vi "Balance_Sweep_Sever.vi"(6 "Mode":bool, 7 "Filename":string, 8 "error in":errorcluster, 9 "Sample Freq (Hz)":dbl=20000.0, 10 "Stop Angle (deg)":dbl=-2.0, 11 "Measurement Time (ms)":u32) -> (0 "error out":errorcluster)   [LabVIEW 2011]
uses:
  Gen Trav/Trav_mode.ctl
  Globals/Trav_pos_global.vi
  Globals/Meas_global.vi
  Controls/Post_Process.ctl
  <userlib>/LV-Link3/PolySubVIs/DtCreateAinChan.vi
  <userlib>/LV-Link3/PolySubVIs/DtOLReadMultiple2D.vi
  <userlib>/LV-Link3/PolySubVIs/DtOLTimingSetInput.vi
  Controls/Live Balance Data.ctl
panel:
  out "status":bool=TRUE
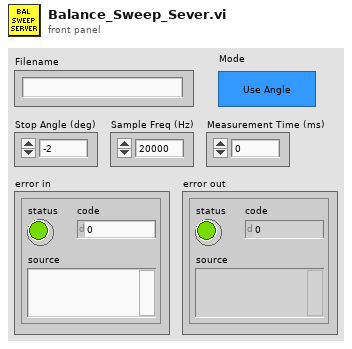
[diagram p1: front panel]
types:
  T1 = typedef "Post_Process.ctl" = enum16{"Take New Data", "Post Process Raw Data File"}
  T2 = typedef "Trav_mode.ctl" = enum16{"Move traverse", "Read traverse position", "Teach Position"}
  T3 = typedef "Live Balance Data.ctl" = cluster{"AS Freq (Hz)":dbl, "Time (s)":dbl[], "Pressure 2 (V)":dbl[], "Pressure 3 (V)":dbl[], "Wind Speed (m/s)":dbl[], "Balance AS Freq (Hz)":dbl[], "Live Angle (deg)":dbl[], "Live Angle An(deg)":dbl[], "Balance Loads":cluster{"Lift (%)":dbl[], "Lift (N)":dbl[], "Pitch (%)":dbl[], "Pitch (Nm)":dbl[], "Drag (%)":dbl[], "Drag (N)":dbl[], "Side (%)":dbl[], "Side (N)":dbl[], "Yaw (%)":dbl[], "Yaw (Nm)":dbl[], "Roll (%)":dbl[], "Roll (Nm)":dbl[]}, "Pressure 1 (V)":dbl[], "Pressure SJ (V)":dbl[]}
  T4 = enum16{"big-endian, network order", "native, host order", "little-endian"}
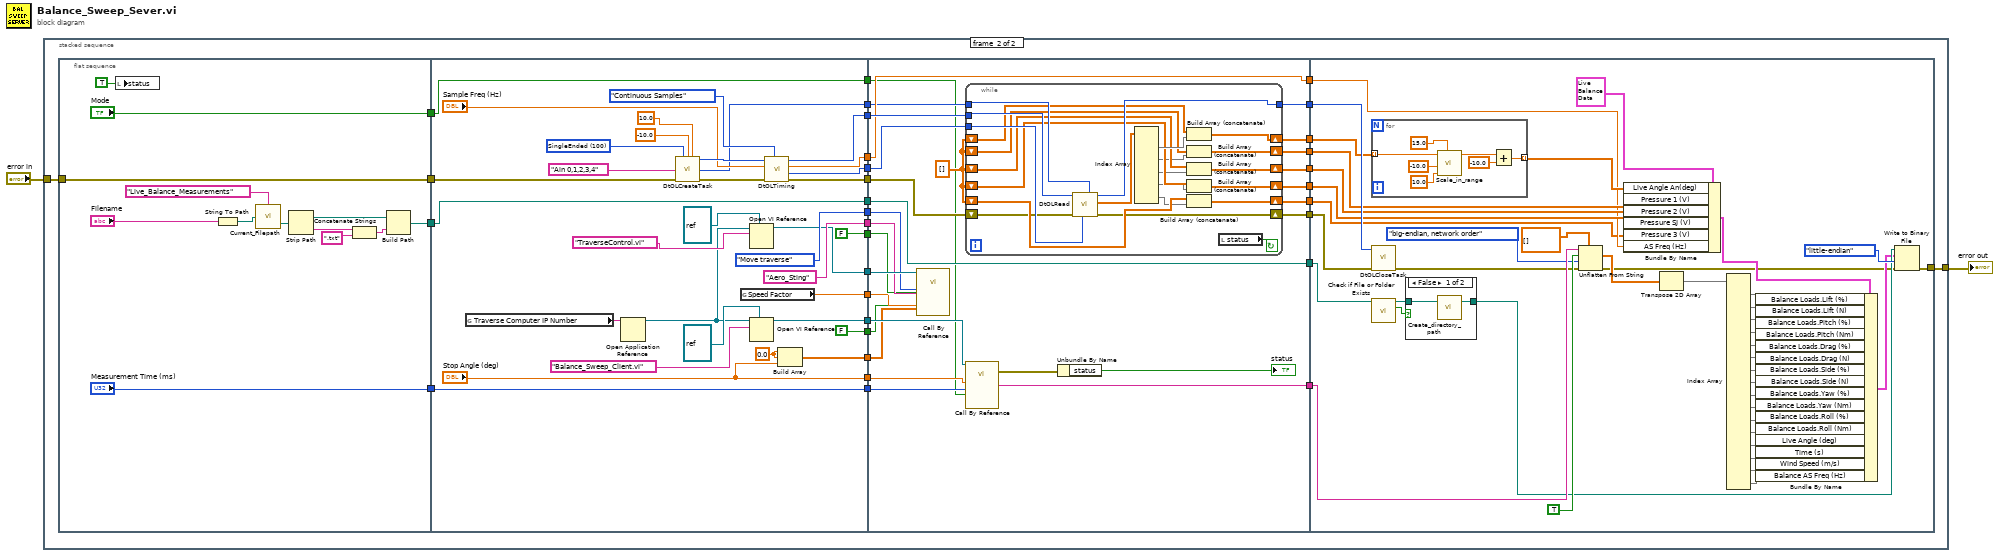
[diagram p0: block diagram]
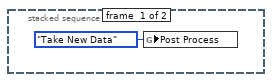
[diagram p2: hidden frame]
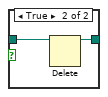
[diagram p3: hidden frame]
diagram:
  n1 = stacked-sequence {
    tunnel: [_ w12] -> w2
    tunnel: "error in" -> [_ w8]
    frame #0 {
      n2 = global write "Meas_global.vi" "Post Process"(Post_Process."Take New Data" ("Post Process")) -> ()
    }
    frame #1 {
      n3 = flat-sequence {
        tunnel: [w45] -> w36
        tunnel: [w39] -> w11
        tunnel: w8 -> [w39]
        tunnel: ["Measurement Time (ms)"] -> w7
        tunnel: ["Mode"] -> w4
        tunnel: [FALSE ("Route Checking?")] -> w35
        tunnel: [Trav_mode."Move traverse" ("Mode")] -> w34
        tunnel: ["Aero_Sting" ("Traverse name")] -> w33
        tunnel: [w78] -> w32
        tunnel: [w76] -> w31
        tunnel: ["Stop Angle (deg)"] -> w30
        tunnel: [w73] -> w29
        tunnel: [w68] -> w28
        tunnel: w36 -> [w73]
        tunnel: [w67] -> w25
        tunnel: [FALSE ("Backlash Compensation?")] -> w24
        tunnel: [w58] -> w23
        tunnel: [w57] -> w22
        tunnel: [w56] -> w20
        tunnel: [w55] -> w19
        tunnel: w11 -> [w54]
        tunnel: [w52] -> w10
        tunnel: w7 -> [w51]
        tunnel: [w51] -> w6
        tunnel: [w50] -> w5
        tunnel: w4 -> [w50]
        tunnel: w35 -> [w102]
        tunnel: w34 -> [w103]
        tunnel: w33 -> [w105]
        tunnel: w32 -> [w104]
        tunnel: w31 -> [w110]
        tunnel: [w109] -> w27
        tunnel: w30 -> [w108]
        tunnel: [w107] -> w26
        tunnel: w29 -> [w107]
        tunnel: w28 -> [w106]
        tunnel: w25 -> [w101]
        tunnel: w24 -> [w100]
        tunnel: w23 -> [w99]
        tunnel: w22 -> [w98]
        tunnel: [w97] -> w21
        tunnel: w20 -> [w97]
        tunnel: w19 -> [w96]
        tunnel: [w95] -> w18
        tunnel: [w93] -> w17
        tunnel: [w92] -> w16
        tunnel: [w91] -> w15
        tunnel: [w90] -> w14
        tunnel: [w88] -> w13
        tunnel: w10 -> [w86]
        tunnel: [w85] -> w9
        tunnel: w6 -> [w84]
        tunnel: w5 -> [w83]
        tunnel: w27 -> [w170]
        tunnel: w26 -> [w175]
        tunnel: w21 -> [w139]
        tunnel: w18 -> [w166]
        tunnel: w17 -> [w141]
        tunnel: w16 -> [w144]
        tunnel: w15 -> [w143]
        tunnel: w14 -> [w142]
        tunnel: w13 -> [w138]
        tunnel: [w137] -> w12
        tunnel: w9 -> [w136]
        frame #0 {
          n4 = local write "status"(TRUE ("status")) -> ()
          n5 = String To Path(string="Filename") -> (path=w47:path)
          n6 = call "Current_Filepath.vi"("Filename in"=w47, "Data Type"="Live_Balance_Measurements") -> ("Filename Out"=w48:path)  [unwired: 1 out]
          n7 = Strip Path(path=w48) -> (stripped path=w41:path, name=w44:string)
          n8 = Concatenate Strings(w44, ".txt" ("string")) -> (w42:string)
          n9 = Build Path(base path=w41, name or relative path=w42) -> (appended path=w45:path)
        }
        frame #1 {
          w62 = 100 items=["SingleEnded"=100, "Differential"=101] ("Channel Type")
          w82 = 0.0
          n10 = global read "Trav_pos_global.vi" "Traverse Computer IP Number"() -> (w72:string)
          n11 = Open Application Reference(11:w72) -> (3:w69:refnum<vi>)  [unwired: 3 in, 1 out]
          n12 = call-poly <userlib>:"DtOLCreateTask.vi"("Channel Type"=w62, "Range Min"=-10.0, "Range Max"=10.0, "Channel"="Ain 0,1,2,3,4", "error in (no error)"=w54) -> ("Task out"=w61:i32, "Actual Number of Channels"=w55:u32, "error out"=w53:errorcluster)  [unwired: 8 in]
          n13 = global read "Trav_pos_global.vi" "Speed Factor"() -> (w67:dbl)
          n14 = Open VI Reference(type specifier VI Refnum (for type only)=refnum<vi> refnum, application reference (local)=w69, vi path="TraverseControl.vi" ("Traverse name")) -> (vi reference=w68:refnum<vi>)  [unwired: 3 in, 1 out]
          n15 = Open VI Reference(type specifier VI Refnum (for type only)=refnum<vi> refnum, application reference (local)=w69, vi path="Balance_Sweep_Client.vi" ("Traverse name")) -> (vi reference=w76:refnum<vi>)  [unwired: 3 in, 1 out]
          n16 = call-poly <userlib>:"DtOLTiming.vi"("Sample Mode"=enum16{"Finite Samples", "Continuous Samples"}."Continuous Samples", "error in (no error)"=w53, "Sample Freq (Hz)"="Sample Freq (Hz)", "Task in"=w61) -> ("error out"=w52:errorcluster, "Buffer Size"=w58:u32, "Actual Sample Freq"=w56:dbl, "Task out"=w57:i32)  [unwired: 4 in]
          n17 = Build Array(w82, w82, "Stop Angle (deg)") -> (w78:dbl[])
        }
        frame #2 {
          w89 = dbl[] []
          n18 = call-by-ref "?"(reference=w106, "Mode"=w103, "Route Checking?"=w102, "Traverse Name"=w105, "Position input XYZ"=w104, "Speed Factor"=w101, "Backlash Compensation?"=w100) -> ()  [unwired: 9 in, 4 out]
          n19 = while {
            tunnel: w99 -> [w133]
            tunnel: w98 -> [w132]
            tunnel: w96 -> [w131]
            tunnel: [w130] -> w95
            shift-right: [w125] -> w93
            shift-left: w89 -> [w126]
            shift-right: [w124] -> w92
            shift-left: w89 -> [w123]
            shift-right: [w121] -> w91
            shift-left: w89 -> [w122]
            shift-right: [w115] -> w90
            shift-left: w89 -> [w120]
            shift-right: [w113] -> w88
            shift-left: w89 -> [w116]
            shift-right: [w111] -> w85
            shift-left: w86 -> [w112]
            stop <- w129 continue-if-true
            n20 = call-poly <userlib>:"DtOLRead.vi"("Number Chan to Read"=w131, "Buffer size"=w133, "error in (no error)"=w112, "Task in"=w132) -> ("error out"=w111:errorcluster, "2D Data out"=w128:dbl[][], "Task out"=w130:i32)  [unwired: 3 in, 2 out]
            n21 = Index Array(array=w128) -> (element #1=w127:dbl[], element #2=w119:dbl[], element #3=w118:dbl[], element #4=w117:dbl[], element #5=w114:dbl[])  [unwired: 10 in]
            n22 = Build Array (concatenate)(w126, w127) -> (w125:dbl[])
            n23 = Build Array (concatenate)(w123, w119) -> (w124:dbl[])
            n24 = Build Array (concatenate)(w122, w118) -> (w121:dbl[])
            n25 = Build Array (concatenate)(w120, w117) -> (w115:dbl[])
            n26 = Build Array (concatenate)(w116, w114) -> (w113:dbl[])
            n27 = local read "status"() -> (w129:bool)
          }
          n28 = call-by-ref "?"(reference=w110, "Mode"=w83, "Measurement Time (ms)"=w84, "Stop Angle"=w108) -> (error out=w94:errorcluster, "Data Out"=w109:string)  [unwired: 3 in, 1 out]
          n29 = Unbundle By Name(w94) -> ("status"=→"status":bool)
        }
        frame #3 {
          n30 = for {
            tunnel: [w179] -> w140 mode=indexing
            tunnel: w141 -> [w176] mode=indexing
            n31 = call "Scale_in_range.vi"("Scale Factor"=15.0, "Maximum Range"=10.0, "Minimum Range"=-10.0, "x"=w176) -> ("Scaled x"=w181:dbl)  [unwired: 7 in]
            n32 = Add(x=w181, y=-10.0) -> (x+y=w179:dbl)
          }
          n33 = call <userlib>:"DtOLCloseTask.vi"("Error in"=w136, "Task in"=w166) -> ("Error Out"=w135:errorcluster)  [unwired: 9 in]
          n34 = call <vilib>:"Check if File or Folder Exists.vi"("path"=w175) -> ("file or folder exists?"=w174:bool, "dup path"=w173:path)  [unwired: 8 in, 1 out]
          n35 = case shown="False" w174 {
            tunnel: w173 -> [w184 w186]
            tunnel: [w183 w185] -> w167
            frame False {
              n36 = call "Create_directory_path.vi"("Path name"=w184) -> ("Path name Out"=w183:path)  [unwired: 1 in, 1 out]
            }
            frame True {
              n37 = Delete(path (use dialog)=w186) -> (deleted path=w185:path)  [unwired: 4 in, 2 out]
            }
          }
          n38 = Unflatten From String(type=dbl[][] [], binary string=w170, data includes array or string size? (T)=TRUE, byte order (0:big-endian, network order)=T4."big-endian, network order", error in (no error)=w135) -> (value=w164:dbl[][], error out=w134:errorcluster)  [unwired: 1 out]
          n39 = Bundle By Name(cluster=T3 {"AS Freq (Hz)"=0.0, "Time (s)"=[], "Pressure 2 (V)"=[], "Pressure 3 (V)"=[], "Wind Speed (m/s)"=[], "Balance AS Freq (Hz)"=[], "Live Angle (deg)"=[], "Live Angle An(deg)"=[], "Balance Loads"={"Lift (%)"=[], "Lift (N)"=[], "Pitch (%)"=[], "Pitch (Nm)"=[], "Drag (%)"=[], "Drag (N)"=[], "Side (%)"=[], "Side (N)"=[], "Yaw (%)"=[], "Yaw (Nm)"=[], "Roll (%)"=[], "Roll (Nm)"=[]}, "Pressure 1 (V)"=[], "Pressure SJ (V)"=[]} ("input cluster"), "Live Angle An(deg)"=w140, "Pressure 1 (V)"=w144, "Pressure 2 (V)"=w143, "Pressure SJ (V)"=w142, "Pressure 3 (V)"=w138, "AS Freq (Hz)"=w139) -> (w163:T3)
          n40 = Transpose 2D Array(2D array=w164) -> (transposed array=w162:dbl[][])
          n41 = Index Array(array=w162) -> (element #1=w160:dbl[], element #2=w159:dbl[], element #3=w158:dbl[], element #4=w157:dbl[], element #5=w156:dbl[], element #6=w155:dbl[], element #7=w154:dbl[], element #8=w153:dbl[], element #9=w152:dbl[], element #10=w151:dbl[], element #11=w150:dbl[], element #12=w149:dbl[], element #13=w148:dbl[], element #14=w147:dbl[], element #15=w146:dbl[], element #16=w145:dbl[])  [unwired: 32 in]
          n42 = Bundle By Name(cluster=w163, "Balance Loads.Lift (%)"=w160, "Balance Loads.Lift (N)"=w159, "Balance Loads.Pitch (%)"=w158, "Balance Loads.Pitch (Nm)"=w157, "Balance Loads.Drag (%)"=w156, "Balance Loads.Drag (N)"=w155, "Balance Loads.Side (%)"=w154, "Balance Loads.Side (N)"=w153, "Balance Loads.Yaw (%)"=w152, "Balance Loads.Yaw (Nm)"=w151, "Balance Loads.Roll (%)"=w150, "Balance Loads.Roll (Nm)"=w149, "Live Angle (deg)"=w148, "Time (s)"=w147, "Wind Speed (m/s)"=w146, "Balance AS Freq (Hz)"=w145) -> (w161:T3)
          n43 = Write to Binary File(file (use dialog)=w167, data=w161, error in=w134, 9:T4."little-endian" ("byte order (0:big-endian, network order)")) -> (error out=w137:errorcluster)  [unwired: 2 in, 2 out]
        }
      }
    }
  }
  "error out" <- w2
